vi "zero_deleter.vi"(1 "Array In":cluster{"X":i32, "Y":i32}[][](array[cluster])) -> (0 "Array Out":cluster{"X":i32, "Y":i32}[][](array[cluster]))   [LabVIEW 2017]
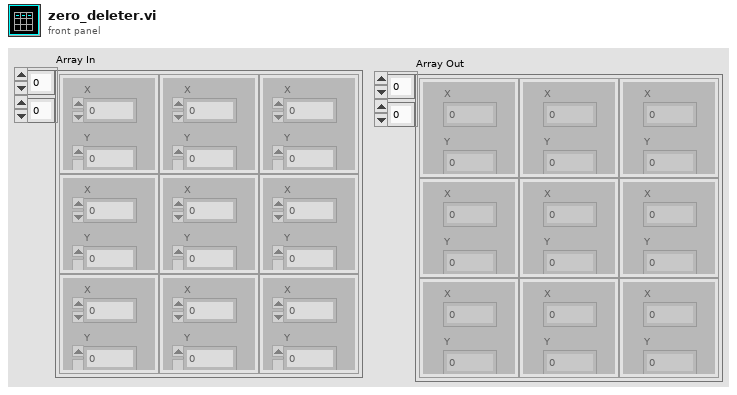
[diagram p1: front panel]
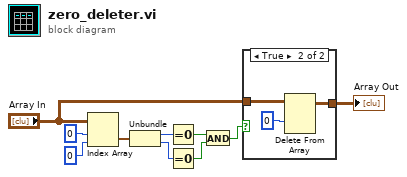
[diagram p0: block diagram]
diagram:
  n1 = Index Array(array="Array In", index (row)=0, index (col)=0 ("disabled index (col)")) -> (element=w7:cluster{"X":i32, "Y":i32})
  n2 = Unbundle(w7) -> ("X"=w4:i32, "Y"=w5:i32)
  n3 = Equal To 0?(x=w4) -> (x = 0?=w2:bool)
  n4 = Equal To 0?(x=w5) -> (x = 0?=w3:bool)
  n5 = And(x=w2, y=w3) -> (x .and. y?=w1:bool)
  n6 = case shown="True" w1 {
    tunnel: "Array In" -> [w11 w14]
    tunnel: [w11 w12] -> w10
    frame False {
    }
    frame True {
      n7 = Delete From Array(array=w14, index (row)=0) -> (array with subset deleted=w12:cluster{"X":i32, "Y":i32}[][])  [unwired: 2 in, 1 out]
    }
  }
  "Array Out" <- w10
